vi "FPGA Main.vi"() -> ()   [LabVIEW 2011]
uses:
  FPGA/TypeDefs/FPGA State.ctl
  Documents/Sales Events/Dev Days 2012/Demos/Demos 2-6/cRIO Fail Safe Ref Design Demo/Storage/Fail-Safe Control FPGA Globals.vi
  <vilib>/rvi/eio/common/nirviEmuTemplateMethod_errors.vi
  FPGA/FPGA Global.vi
  <vilib>/eio/EIONode/EIONode.xnode
panel:
  out "pH":fxp<+/-,20,5> format="%.17g"
  out "Temp Data":fxp<+/-,24,-2>[](array[numeric]) format="%.26g"
  out "Emergency Stop":bool
  in  "PWM Duty Cycle (Ticks)":i32
  out "FPGA State":T1
  in  "Update Period(uSec)":u32=100000 caption="Count(uSec)"
  in  "Waste":bool
  in  "Intake":bool
  in  "Acid":bool
  in  "Heater":bool
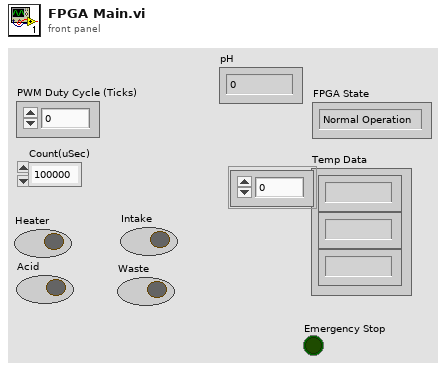
[diagram p1: front panel]
types:
  T1 = typedef "FPGA State.ctl" = enum16{"Normal Operation", "Safe State"}
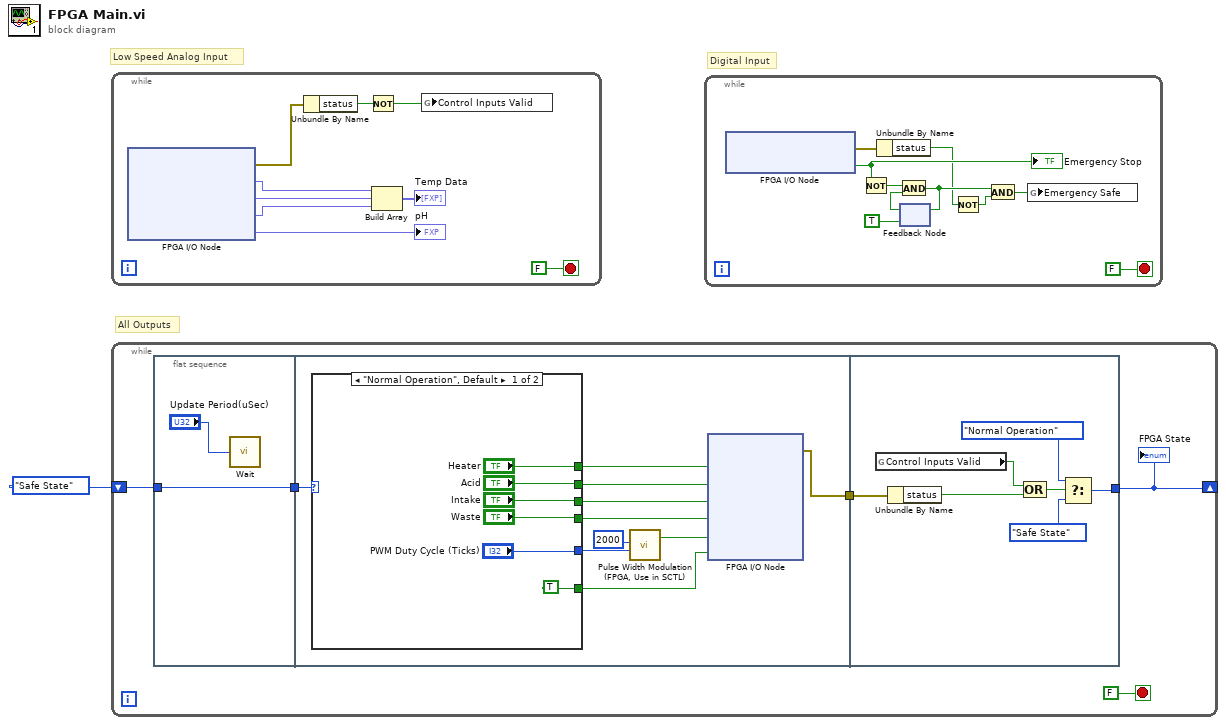
[diagram p0: block diagram]
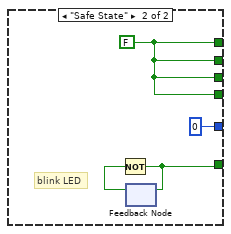
[diagram p2: hidden frame]
diagram:
  # "Digital Input"
  # "All Outputs"
  # "Low Speed Analog Input"
  n1 = while {
    stop <- FALSE stop-if-true
    n2 = xnode "FPGA I/O Node"() -> ("error out"=w9:errorcluster, "Temp/TC0"=w6:fxp<+/-,24,-2>, "Temp/CJC"=w5:fxp<+/-,24,-2>, "Temp/Autozero"=w4:fxp<+/-,24,-2>, "pH"=→"pH":fxp<+/-,20,5>)  [unwired: 5 in, 4 out]
    n3 = Unbundle By Name(w9) -> ("status"=w8:bool)
    n4 = Not(x=w8) -> (.not. x?=w7:bool)
    n5 = Build Array(w6, w5, w4) -> (→"Temp Data":fxp<+/-,24,-2>[])
    n6 = global write "FPGA Global.vi" "Control Inputs Valid"(w7) -> ()
  }
  n7 = while {
    shift-right: [w12] -> _
    shift-left: FPGA_State."Safe State" -> [w11]
    stop <- FALSE stop-if-true
    n8 = flat-sequence {
      tunnel: w11 -> [w17]
      tunnel: [w17] -> w14
      tunnel: w14 -> [w27]
      tunnel: [w22] -> w13
      tunnel: w13 -> [w43]
      tunnel: [w38] -> w12
      frame #0 {
        n9 = call "Wait"("Count(uSec)"="Update Period(uSec)") -> ()  [unwired: 1 out]
      }
      frame #1 {
        n10 = case shown="\"Normal Operation\", Default" w27 {
          tunnel: ["Heater" w36] -> w26
          tunnel: ["Acid" w36] -> w25
          tunnel: ["Intake" w36] -> w24
          tunnel: ["Waste" w36] -> w23
          tunnel: [TRUE w35] -> w21
          tunnel: ["PWM Duty Cycle (Ticks)" 0 ("PWM Duty Cycle (Ticks)")] -> w18
          frame "Normal Operation", Default {
          }
          frame "Safe State" {
            w36 = FALSE
            # "blink LED"
            n11 = feedback #1() -> (w37:bool)  [unwired: 1 in]
            n12 = Not(x=w37) -> (.not. x?=w35:bool)
            n13 = feedback-in #1(w35) -> ()
          }
        }
        n14 = call "Pulse Width Modulation (FPGA, Use in SCTL).vi"("PWM Period (Ticks)"=u32 2000, "PWM Duty Cycle (Ticks)"=w18) -> ("PWM DO"=w20:bool)  [unwired: 12 in, 5 out]
        n15 = xnode "FPGA I/O Node"("Heater"=w26, "Acid"=w25, "Intake"=w24, "Waste"=w23, "Agitator"=w20, "FPGA LED"=w21) -> ("error out"=w22:errorcluster)  [unwired: 7 in, 6 out]
      }
      frame #2 {
        n16 = global read "FPGA Global.vi" "Control Inputs Valid"() -> (w44:bool)
        n17 = Unbundle By Name(w43) -> ("status"=w42:bool)
        n18 = Compound Arithmetic op=OR(w44, w42) -> (w41:bool)
        n19 = Select(t=FPGA_State."Normal Operation", s=w41, f=FPGA_State."Safe State") -> (s? t:f=w38:T1)
      }
    }
    "FPGA State" <- w12
  }
  n20 = while {
    stop <- FALSE stop-if-true
    n21 = xnode "FPGA I/O Node"() -> ("error out"=w46:errorcluster, "Emergency Stop"=w48:bool)  [unwired: 2 in, 1 out]
    "Emergency Stop" <- w48
    n22 = Not(x=w48) -> (.not. x?=w51:bool)
    n23 = Unbundle By Name(w46) -> ("status"=w45:bool)
    n24 = feedback #2(TRUE) -> (w53:bool)
    n25 = And(x=w51, y=w53) -> (x .and. y?=w47:bool)
    n26 = feedback-in #2(w47) -> ()
    n27 = Not(x=w45) -> (.not. x?=w50:bool)
    n28 = And(x=w47, y=w50) -> (x .and. y?=w49:bool)
    n29 = global write "Fail-Safe Control FPGA Globals.vi" "Emergency Safe"(w49) -> ()
  }
